vi "Destroy.vi"(0 "reference in":refnum<class "Data Generator.lvclass">, 11 "Error In":errorcluster) -> (4 "reference out":refnum<class "Data Generator.lvclass">, 15 "Error Out":errorcluster)   [LabVIEW 2024, in "Data Generator.lvclass"]
uses:
  Data Generator.lvclass
  Data Generator.lvclass/Data Generator.ctl
panel:
  # "Connector Pane"
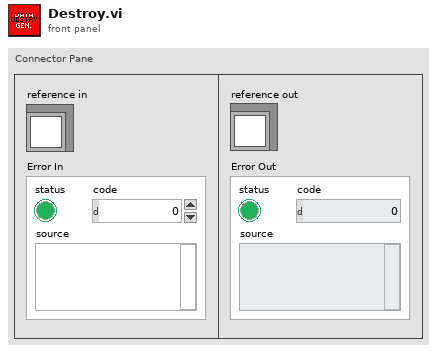
[diagram p1: front panel]
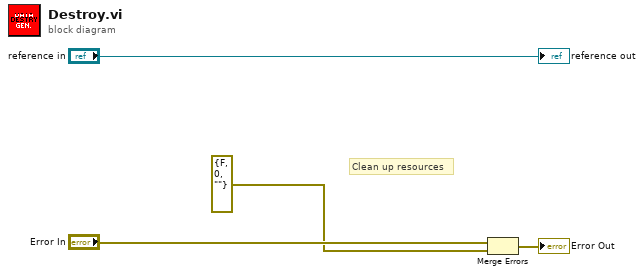
[diagram p0: block diagram]
diagram:
  # "Clean up resources"
  n1 = Merge Errors("Error In", errorcluster {"status"=FALSE, "code"=0, "source"=""} ("error in")) -> (→"Error Out":errorcluster)
  "reference out" <- "reference in"
